vi "Record.vi"(6 "Last request":bool, 8 "error in (no error)":errorcluster, 11 "Spectrum Recorder in":refnum<class "Spectrum Recorder too.lvclass">) -> (0 "error out":errorcluster, 2 "Result":refnum<class "Acquired Result.lvclass">, 3 "Spectrum Recorder out":refnum<class "Spectrum Recorder too.lvclass">)   [LabVIEW 2016, in "Spectrum Recorder too.lvclass"]
uses:
  Spectrum Recorder too.lvclass
  C:/github/LabActor/Worker/Worker.lvclass
  C:/github/LabActor/Instrument Actor/Instrument Actor.lvclass
  NHMFL_Core/Libraries/Instruments/Results/Acquired Result/Acquired Result.lvclass
  Worker/Worker.lvclass/Worker.ctl
  Spectrum Recorder too.lvclass/Spectrum Recorder too.ctl
  Template Module/Read State.vi
  Read RP transceiver.vi
  Write RP transceiver.vi
  NHMFL_Core/Libraries/Red Pitaya/RP Core/RP Transceiver/RP Transceiver.lvclass
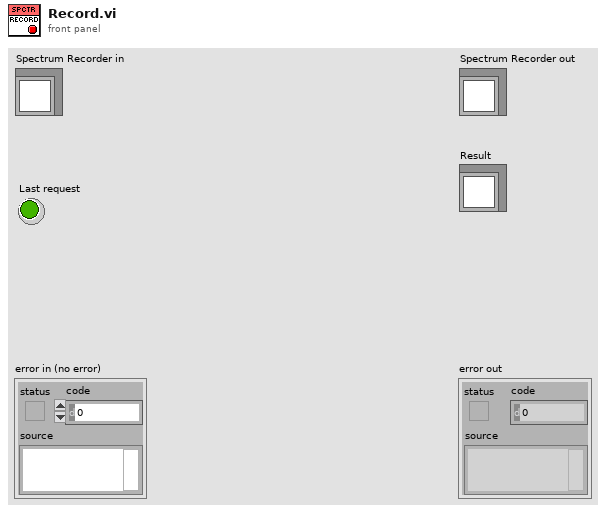
[diagram p1: front panel]
types:
  T1 = typedef "Worker State.ctl" = enum16{"Idle", "Starting", "Working", "Stopping"}
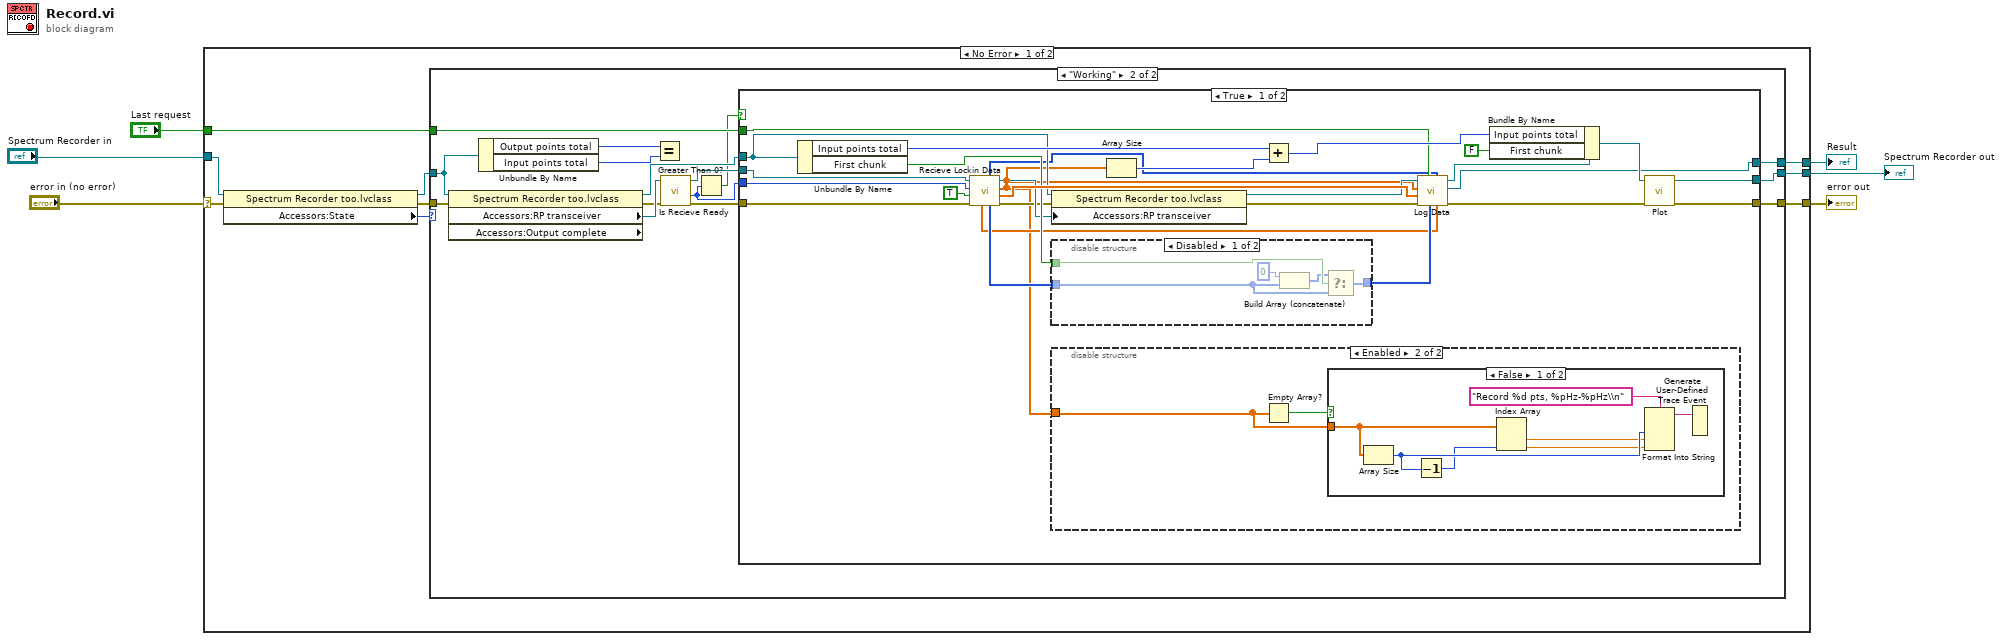
[diagram p0: block diagram]
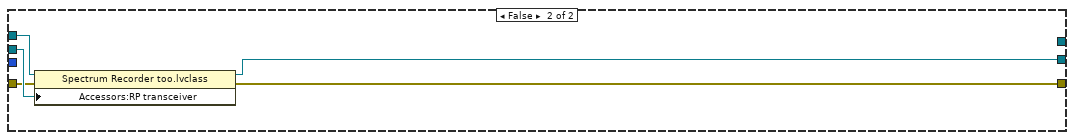
[diagram p6: hidden frame]
diagram:
  n1 = case shown="No Error" "error in (no error)" {
    selector: "error in (no error)" -> [w14 w81]
    tunnel: [w13 w81] -> w5
    tunnel: [w15 w80] -> w3
    tunnel: "Spectrum Recorder in" -> [w11 w80]
    tunnel: "Last request" -> [w8 _]
    tunnel: [w7 _] -> w1
    frame No Error {
      n2 = property class="Spectrum Recorder too.lvclass"(reference=w11, error in=w14) -> (reference out=w10:refnum<class "Spectrum Recorder too.lvclass">, error out=w12:errorcluster, "Accessors:State"=w9:T1)
      n3 = case shown="\"Working\"" w9 {
        tunnel: w10 -> [w17 w24]
        tunnel: w12 -> [w16 w27]
        tunnel: [w17 w29] -> w15
        tunnel: [w16 w30] -> w13
        tunnel: w8 -> [_ w20]
        tunnel: [_ w19] -> w7
        frame "Idle", Default {
        }
        frame "Working" {
          n4 = property class="Spectrum Recorder too.lvclass" props=["Accessors:RP transceiver", "Accessors:Output complete"](reference=w24, error in=w27) -> (reference out=w25:refnum<class "Spectrum Recorder too.lvclass">, error out=w26:errorcluster, "Accessors:RP transceiver"=w28:refnum<class "RP Transceiver.lvclass">)  [unwired: 1 out]
          n5 = Unbundle By Name(w24) -> ("Output points total"=w23:i64, "Input points total"=w22:i64)
          n6 = Equal?(x=w23, y=w22) -> ()  [unwired: 1 out]
          n7 = call-dynamic "Is Recieve Ready.vi"("error in (no error)"=w26, "RP Instrument in"=w28) -> ("error out"=w32:errorcluster, "Points in buffer"=w21:i32, "RP Instrument out"=w31:refnum<class "RP Transceiver.lvclass">)  [unwired: 6 in, 1 out]
          n8 = Greater Than 0?(x=w21) -> (x > 0?=w18:bool)
          n9 = case shown="True" w18 {
            tunnel: w32 -> [w59 w75]
            tunnel: w31 -> [w58 w76]
            tunnel: w21 -> [w57 _]
            tunnel: [w49 w78] -> w30
            tunnel: [w47 w79] -> w29
            tunnel: w25 -> [w43 w77]
            tunnel: w20 -> [w38 _]
            tunnel: [w35 _] -> w19
            frame True {
              n10 = Unbundle By Name(w43) -> ("Input points total"=w44:i64, "First chunk"=w55:bool)
              n11 = call-dynamic "Recieve Lockin Data.vi"("error in (no error)"=w59, "Force read"=TRUE, "Points to read"=w57, "RP Lockin in"=w58) -> ("error out"=w39:errorcluster, "Volatge X out"=w56:dbl[], "Frequency out"=w33:dbl[], "RP Lockin out"=w40:refnum<class "RP Transceiver.lvclass">, "Starting edges"=w50:i32[], "Ending edges"=w37:i32[], "Volatge Y out"=w36:dbl[])  [unwired: 1 in]
              n12 = property class="Spectrum Recorder too.lvclass"(reference=w43, error in=w39, "Accessors:RP transceiver"=w40) -> (reference out=w42:refnum<class "Spectrum Recorder too.lvclass">, error out=w41:errorcluster)
              n13 = disable-structure shown="Disabled" {
                disable-tunnel: w55 -> [w73 _]
                disable-tunnel: [w70 w74] -> w54
                disable-tunnel: w50 -> [w69 w74]
                frame Disabled {
                  n14 = Build Array (concatenate)(0, w69) -> (w71:i32[])
                  n15 = Select(t=w71, s=w73, f=w69) -> (s? t:f=w70:i32[])
                }
                frame Enabled {
                }
              }
              n16 = disable-structure shown="Enabled" {
                disable-tunnel: w33 -> [_ w60]
                frame Disabled {
                }
                frame Enabled {
                  n17 = Empty Array?(array=w60) -> (empty?=w61:bool)
                  n18 = case shown="False" w61 {
                    tunnel: w60 -> [w67 _]
                    frame False {
                      n19 = Array Size(array=w67) -> (size(s)=w66:i32)
                      n20 = Decrement(x=w66) -> (x-1=w65:i32)
                      n21 = Index Array(array=w67, index #2=w65) -> (element #1=w64:dbl, element #2=w63:dbl)  [unwired: 1 in]
                      n22 = Format Into String(format string="Record %d pts, %pHz-%pHz\\n", w66, w64, w63) -> (resulting string=w62:string)  [unwired: 2 in, 1 out]
                      n23 = Generate User-Defined Trace Event(2:w62) -> ()  [unwired: 1 in]
                    }
                    frame True {
                    }
                  }
                }
              }
              n24 = Array Size(array=w33) -> (size(s)=w45:i32)
              n25 = Add(x=w44, y=w45) -> (x+y=w46:i64)
              n26 = call-dynamic "Log Data.vi"("Volatge Y"=w36, "Ending edges"=w37, "Starting edges"=w54, "Last request"=w38, "error in (no error)"=w41, "Volatge X"=w56, "Frequency"=w33, "Spectrum Recorder in"=w42) -> ("error out"=w52:errorcluster, "Result"=w35:refnum<class "Acquired Result.lvclass">, "Spectrum Recorder out"=w53:refnum<class "Spectrum Recorder too.lvclass">)  [unwired: 1 in]
              n27 = Bundle By Name(cluster=w53, "Input points total"=w46, "First chunk"=FALSE) -> (w48:refnum<class "Spectrum Recorder too.lvclass">)
              n28 = call-dynamic "Plot.vi"("error in (no error)"=w52, "Spectrum Recorder in"=w48) -> ("error out"=w49:errorcluster, "Spectrum Recorder out"=w47:refnum<class "Spectrum Recorder too.lvclass">)  [unwired: 8 in]
            }
            frame False {
              n29 = property class="Spectrum Recorder too.lvclass"(reference=w77, error in=w75, "Accessors:RP transceiver"=w76) -> (reference out=w79:refnum<class "Spectrum Recorder too.lvclass">, error out=w78:errorcluster)
            }
          }
        }
      }
    }
    frame Error {
    }
  }
  "error out" <- w5
  "Spectrum Recorder out" <- w3
  "Result" <- w1
